vi "ChirpMeasurementV2.vi"(8 "error in (no error)":errorcluster, 11 "ChirpV2 in":refnum<class "ChirpV2.lvclass">) -> (0 "error out":errorcluster, 1 "Duration":dbl, 2 "data 3":dynamicdata(graph) caption="data", 3 "ChirpV2 out":refnum<class "ChirpV2.lvclass">)   [LabVIEW 2014, in "ChirpV2.lvclass"]
uses:
  ChirpV2.lvclass
  <vilib>/Analysis/4window.llb/Cosine Tapered Window (DBL).vi
  <vilib>/measure/NI_MABase.lvlib
  <vilib>/addons/_NISVFA/_Generation/SoundVib_Generation.lvlib
  <vilib>/Analysis/NI_AALPro.lvlib
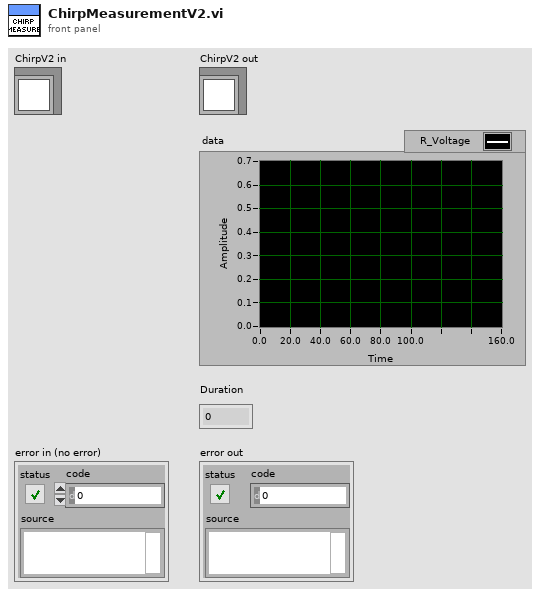
[diagram p1: front panel]
types:
  T1 = cluster{"start frequency [Hz]":dbl, "stop frequency [Hz]":dbl}
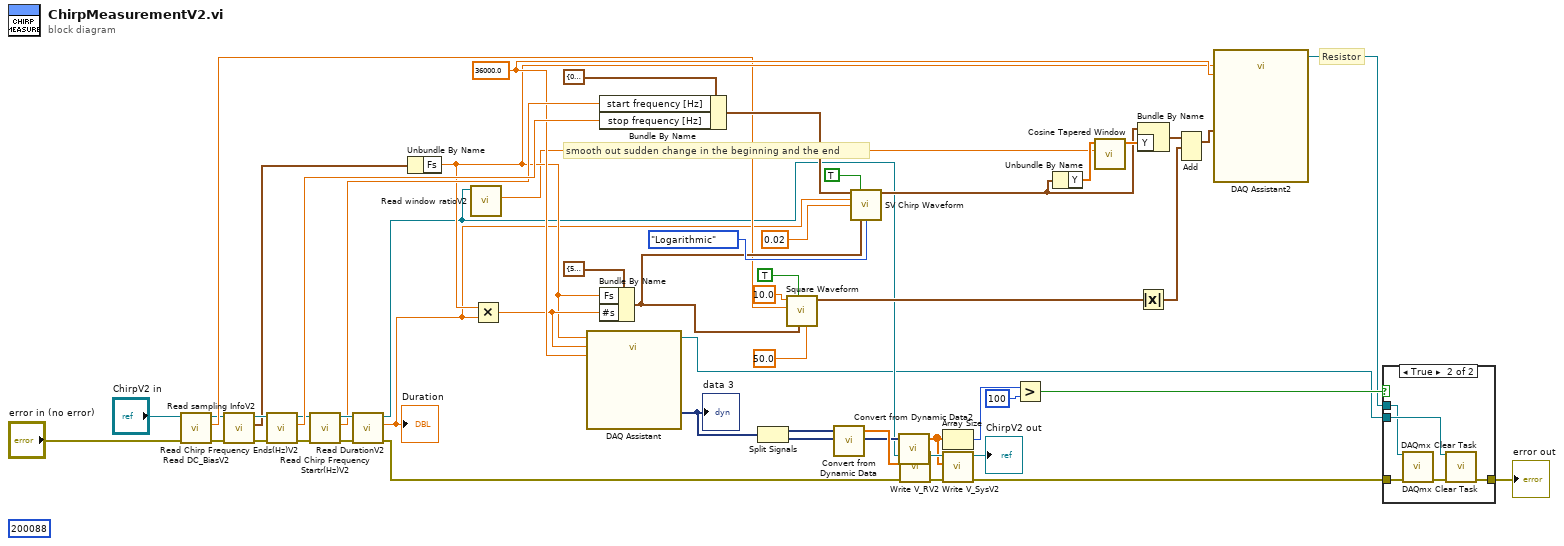
[diagram p0: block diagram]
diagram:
  (unwired) 200088 ("specific error code to clear (0: all)")
  w29 = 36000.0 ("timeout (s)")
  # "smooth out sudden change in the beginning and the end"
  # "Resistor"
  n1 = call-dynamic "Read DC_BiasV2.vi"("error in (no error)"="error in (no error)", "ChirpV2 in"="ChirpV2 in") -> ("error out"=w17:errorcluster, "DC_Bias"=w18:dbl, "ChirpV2 out"=w16:refnum<class "ChirpV2.lvclass">)  [unwired: 7 in]
  n2 = call-dynamic "Read sampling InfoV2.vi"("error in (no error)"=w17, "ChirpV2 in"=w16) -> ("error out"=w43:errorcluster, "sampling Info"=w19:cluster{"Fs":dbl}, "ChirpV2 out"=w38:refnum<class "ChirpV2.lvclass">)  [unwired: 7 in]
  n3 = call-dynamic "Read Chirp Frequency Ends(Hz)V2.vi"("error in (no error)"=w43, "ChirpV2 in"=w38) -> ("error out"=w44:errorcluster, "Chirp Frequency Ends(Hz)"=w42:dbl, "ChirpV2 out"=w39:refnum<class "ChirpV2.lvclass">)  [unwired: 7 in]
  n4 = call-dynamic "Read Chirp Frequency Startr(Hz)V2.vi"("error in (no error)"=w44, "ChirpV2 in"=w39) -> ("error out"=w47:errorcluster, "Chirp Frequency Startr(Hz)"=w41:dbl, "ChirpV2 out"=w46:refnum<class "ChirpV2.lvclass">)  [unwired: 7 in]
  n5 = call-dynamic "Read DurationV2.vi"("error in (no error)"=w47, "ChirpV2 in"=w46) -> ("error out"=w48:errorcluster, "Duration"=w11:dbl, "ChirpV2 out"=w10:refnum<class "ChirpV2.lvclass">)  [unwired: 7 in]
  "Duration" <- w11
  n6 = Unbundle By Name(w19) -> ("Fs"=w27:dbl)
  n7 = call-dynamic "Read window ratioV2.vi"("ChirpV2 in"=w10) -> ("window ratio"=w9:dbl)  [unwired: 8 in, 2 out]
  n8 = Multiply(x=w27, y=w11) -> (x*y=w28:dbl)
  n9 = call "DAQ Assistant"("rate"=w27, "number of samples"=w28, "timeout (s)"=w29) -> ("task out"=w4:refnum<k21>, "data"=w32:dynamicdata)  [unwired: 14 in, 1 out]
  "data 3" <- w32
  n10 = Bundle By Name(cluster=T1 {"start frequency [Hz]"=0.01, "stop frequency [Hz]"=10.0} ("frequency range"), "start frequency [Hz]"=w41, "stop frequency [Hz]"=w42) -> (w45:T1)
  n11 = Bundle By Name(cluster=cluster{"Fs":dbl, "#s":u32} {"Fs"=51200.0, "#s"=1024} ("sampling info"), "Fs"=w27, "#s"=w28) -> (w21:cluster{"Fs":dbl, "#s":u32})
  n12 = Split Signals(w32) -> (w30:dynamicdata, w31:dynamicdata)  [unwired: 2 in]
  n13 = call <vilib>:"Square Waveform.vi"("duty cycle (%)"=50.0, "sampling info"=w21, "reset signal"=TRUE, "amplitude"=w18, "frequency"=10.0) -> ("signal out"=w14:waveform(dbl))  [unwired: 5 in, 1 out]
  n14 = call "Convert from Dynamic Data"("Dynamic Data Type"=w30) -> ("Array"=w33:dbl[])  [unwired: 3 in]
  n15 = call <vilib>:"SV Chirp Waveform.vi"("frequency range"=w45, "reset signal (F)"=TRUE, "chirp duration [s]"=w11, "amplitude"=0.02, "sampling info"=w21, "frequency spacing"=enum16{"Linear", "Logarithmic"}."Logarithmic") -> ("chirp signal"=w49:waveform(dbl))  [unwired: 7 in, 2 out]
  n16 = call "Convert from Dynamic Data2"("Dynamic Data Type"=w31) -> ("Array"=w3:dbl[])  [unwired: 3 in]
  n17 = call-dynamic "Write V_RV2.vi"("error in (no error)"=w48, "V_R"=w33, "ChirpV2 in"=w10) -> ("error out"=w35:errorcluster, "ChirpV2 out"=w34:refnum<class "ChirpV2.lvclass">)  [unwired: 7 in]
  n18 = Array Size(array=w3) -> (size(s)=w8:i32)
  n19 = call-dynamic "Write V_SysV2.vi"("error in (no error)"=w35, "V_Sys"=w3, "ChirpV2 in"=w34) -> ("error out"=w2:errorcluster, "ChirpV2 out"=→"ChirpV2 out":refnum<class "ChirpV2.lvclass">)  [unwired: 7 in]
  n20 = Greater?(x=w8, y=100) -> (0:w7:bool)
  n21 = Unbundle By Name(w49) -> ("Y"=w50:dbl[])
  n22 = call-poly <vilib>:"Cosine Tapered Window.vi"("ratio"=w9, "X"=w50) -> ("Windowed X"=w51:dbl[])  [unwired: 8 in, 1 out]
  n23 = Bundle By Name(cluster=w49, "Y"=w51) -> (w52:waveform(dbl))
  n24 = Absolute Value(x=w14) -> (abs(x)=w23:waveform(dbl))
  n25 = Add(1:w23, 2:w52) -> (0:w24:waveform(dbl))  [unwired: 1 in, 1 out]
  n26 = call "DAQ Assistant2"("data"=w24, "rate"=w27, "timeout (s)"=w29) -> ("task out"=w5:refnum<k21>)  [unwired: 14 in, 2 out]
  n27 = case shown="True" w7 {
    tunnel: w5 -> [_ w58]
    tunnel: w4 -> [_ w59]
    tunnel: w2 -> [w54 w57]
    tunnel: [w54 w55] -> w1
    frame False {
    }
    frame True {
      n28 = call <vilib>:"DAQmx Clear Task.vi"("task in"=w58, "error in"=w57) -> ("error out"=w56:errorcluster)  [unwired: 13 in]
      n29 = call <vilib>:"DAQmx Clear Task.vi"("task in"=w59, "error in"=w56) -> ("error out"=w55:errorcluster)  [unwired: 13 in]
    }
  }
  "error out" <- w1
